vi "Write Peak Field.vi"(8 "error in (no error)":errorcluster, 10 "Peak Field":dbl, 11 "Monitor-Pulse in":refnum<class "Monitor-Pulse.lvclass">) -> (0 "error out":errorcluster, 3 "Monitor-Pulse out":refnum<class "Monitor-Pulse.lvclass">)   [LabVIEW 2015, in "Monitor-Pulse.lvclass"]
uses:
  Monitor-Pulse.lvclass
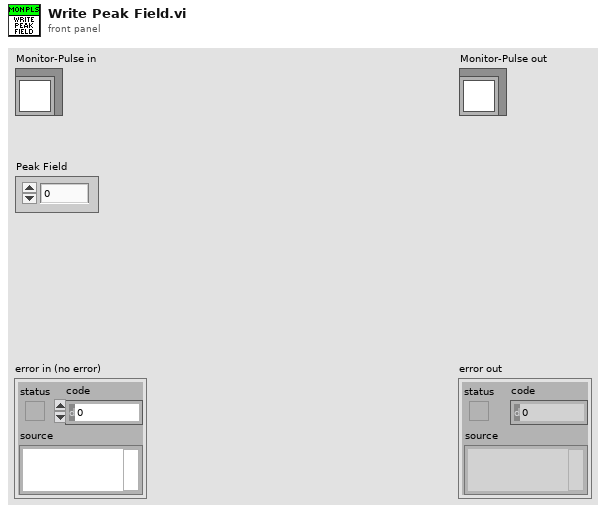
[diagram p1: front panel]
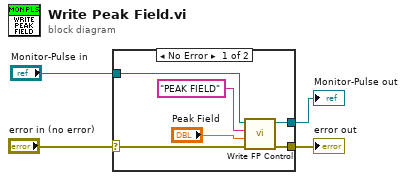
[diagram p0: block diagram]
diagram:
  n1 = case shown="No Error" "error in (no error)" {
    selector: "error in (no error)" -> [w6 w12]
    tunnel: [w5 w12] -> w3
    tunnel: [w9 w11] -> w1
    tunnel: "Monitor-Pulse in" -> [w10 w11]
    frame No Error {
      n2 = call-dynamic "Write FP Control.vi"("error in (no error)"=w6, "Control Value"="Peak Field", "Control Name"="PEAK FIELD", "Measure Object in"=w10) -> ("error out"=w5:errorcluster, "Measure Object out"=w9:refnum<class "Monitor-Pulse.lvclass">)  [unwired: 6 in]
    }
    frame Error {
    }
  }
  "error out" <- w3
  "Monitor-Pulse out" <- w1
